vi "Sample--ContSave.vi"() -> ()   [LabVIEW 2013]
doc: "This samples demonstrates how to sample a finite waveform."
uses:
  <userlib>/ArtScope/Trigger/ArtScope_ConfigureTriggerSoftWare.vi
  <userlib>/ArtScope/Fetch/ArtScope_FetchBinary8.vi
  <userlib>/ArtScope/_SubVI/ArtScope_ArrayByChannel_U8.vi
panel:
  out "error out":errorcluster
  in  "reference position":dbl
  in  "range(Vpp)":i32(ring) items=["20V", "10V", "2V", "40V", "16V", "8V", "4V", "1.6V", "800m", "400m", "160m", "80m", "40m"]
  in  "Stop":bool
  out "波形图":u8[][](graph)
  in  "FileName":string="D:\\1.PCI"
  in  "MinRecordLength":i32=60000
  in  "MinSampleRate":dbl=800000.0
  in  "Coupling":i32(ring) items=["DC", "AC"]
  in  "Channel Name":string="0"
  in  "resource name":string="Dev2"
  # "Vertical"
  # "Horizontal"
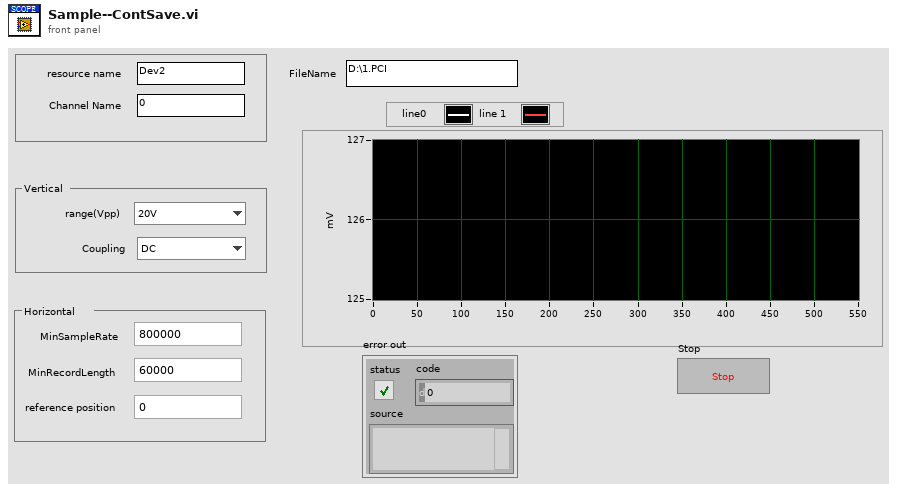
[diagram p1: front panel]
types:
  T1 = cluster{"fLSB":cluster{dbl, dbl, dbl, dbl, dbl, dbl, dbl, dbl}, "RangeValue":cluster{dbl, dbl, dbl, dbl, dbl, dbl, dbl, dbl}, "wMaxLSB":u32, "TriggerMode":i32, "sampLengthPerChan":u32, "pAvailSampsPoints":u32, "channelCount":i32}
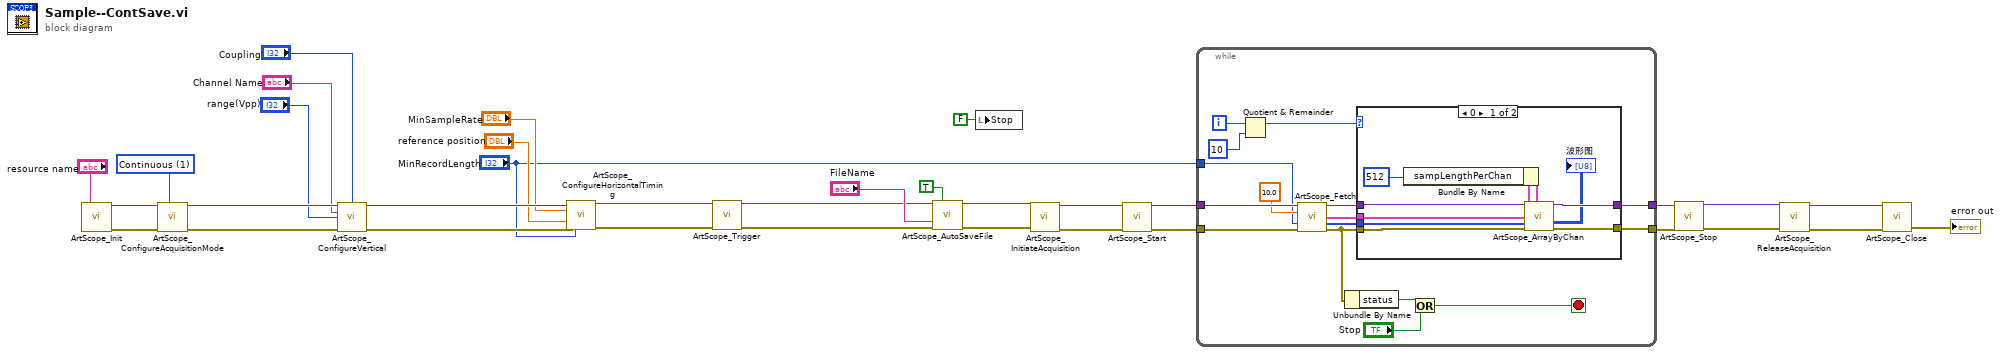
[diagram p0: block diagram]
diagram:
  w26 = 1 items=["Finite", "Continuous"] ("AcuqMode")
  n1 = call <userlib>:"ArtScope_Init.vi"("task name"="resource name") -> ("task handle"=w27:variant, "error out"=w28:errorcluster)  [unwired: 13 in]
  n2 = call <userlib>:"ArtScope_ConfigureAcquisitionMode.vi"("task handle"=w27, "acquisition mode"=w26, "error in (no error)"=w28) -> ("task handle"=w25:variant, "error out"=w29:errorcluster)  [unwired: 11 in]
  n3 = call <userlib>:"ArtScope_ConfigureVertical.vi"("task handle"=w25, "coupling"="Coupling", "channels"="Channel Name", "range(Vpp)"="range(Vpp)", "error in (no error)"=w29) -> ("task handle"=w31:variant, "error out"=w30:errorcluster)  [unwired: 9 in]
  n4 = call <userlib>:"ArtScope_ConfigureHorizontalTiming.vi"("task handle"=w31, "min sample rate"="MinSampleRate", "reference position"="reference position", "error in (no error)"=w30, "min record length"="MinRecordLength") -> ("task handle"=w23:variant, "error out"=w24:errorcluster)  [unwired: 9 in]
  n5 = call-poly <userlib>:"ArtScope_Trigger.vi"("task handle"=w23, "error in (no error)"=w24) -> ("task handle"=w13:variant, "error out"=w12:errorcluster)  [unwired: 12 in]
  n6 = call <userlib>:"ArtScope_AutoSaveFile.vi"("task handle"=w13, "auto save"=TRUE ("AutoSave"), "file name"="FileName", "error in (no error)"=w12) -> ("task handle"=w10:variant, "error out"=w11:errorcluster)  [unwired: 10 in]
  n7 = local write "Stop"(FALSE ("停止")) -> ()
  n8 = call <userlib>:"ArtScope_InitiateAcquisition.vi"("task handle"=w10, "error in (no error)"=w11) -> ("task handle"=w19:variant, "error out"=w18:errorcluster)  [unwired: 12 in]
  n9 = call <userlib>:"ArtScope_Start.vi"("task handle"=w19, "error in (no error)"=w18) -> ("task handle"=w6:variant, "error out"=w5:errorcluster)  [unwired: 12 in]
  n10 = while {
    tunnel: [w35] -> w8
    tunnel: [w36] -> w7
    tunnel: w6 -> [w50]
    tunnel: w5 -> [w49]
    tunnel: "MinRecordLength" -> [w41]
    i -> [w44]
    stop <- w47 stop-if-true
    n11 = Quotient & Remainder(x=w44, y=10) -> (x-y*floor(x/y)=w42:i32)  [unwired: 1 out]
    n12 = call-poly <userlib>:"ArtScope_Fetch.vi"("task handle"=w50, "timeout"=10.0 ("Timeout(s)"), "num samples"=w41, "error in (no error)"=w49) -> ("task handle"=w40:variant, "wfm info"=w38:T1, "data"=w37:u8[], "error out"=w39:errorcluster)  [unwired: 8 in]
    n13 = Unbundle By Name(w39) -> ("status"=w46:bool)
    n14 = case shown="0" w42 {
      tunnel: w40 -> [w59 w61]
      tunnel: w39 -> [w58 w60]
      tunnel: w38 -> [w56 _]
      tunnel: w37 -> [w57 _]
      tunnel: [w53 w61] -> w36
      tunnel: [w52 w60] -> w35
      frame 0 {
        n15 = Bundle By Name(cluster=w56, "sampLengthPerChan"=u32 512 ("Length")) -> (w54:T1)
        n16 = call-poly <userlib>:"ArtScope_ArrayByChan.vi"("task handle"=w59, "wfm info"=w54, "1D data"=w57, "error in (no error)"=w58) -> ("task handle"=w53:variant, "2D data"=→"波形图":u8[][], "error out"=w52:errorcluster)  [unwired: 9 in]
      }
      frame 1, Default {
      }
    }
    n17 = Or(x=w46, y="Stop") -> (x .or. y?=w47:bool)
  }
  n18 = call <userlib>:"ArtScope_Stop.vi"("task handle"=w7, "error in (no error)"=w8) -> ("task handle"=w17:variant, "error out"=w16:errorcluster)  [unwired: 12 in]
  n19 = call <userlib>:"ArtScope_ReleaseAcquisition.vi"("task handle"=w17, "error in (no error)"=w16) -> ("task handle"=w15:variant, "error out"=w14:errorcluster)  [unwired: 12 in]
  n20 = call <userlib>:"ArtScope_Close.vi"("task handle"=w15, "error in (no error)"=w14) -> ("error out"=→"error out":errorcluster)  [unwired: 13 in]
